vi "Media整体图.vi"() -> ()   [LabVIEW 2014]
panel:
  in  "Mute":bool
  in  "Music":bool
  in  "Multimedia":bool
  in  "Mix":bool
  in  "Mediaplayer":bool
  in  "Jukebox":bool
  in  "Ipod":bool
  in  "Dvd":bool
  in  "Create":bool
  in  "Control":bool
  in  "Chat":bool
  in  "Cdwriter":bool
  in  "Cdrom":bool
  in  "Cd":bool
  in  "Camera":bool
  in  "Build":bool
  in  "Bell":bool
  in  "Audio cd":bool
  in  "Arts":bool
  in  "Action":bool
  in  "Volume":bool
  in  "Unknown":bool
  in  "Tv":bool
  in  "Sound":bool
  in  "Snap":bool
  in  "Record volume":bool
  in  "Realplayer":bool
  in  "Player":bool
  in  "Play":bool
  in  "Piano":bool
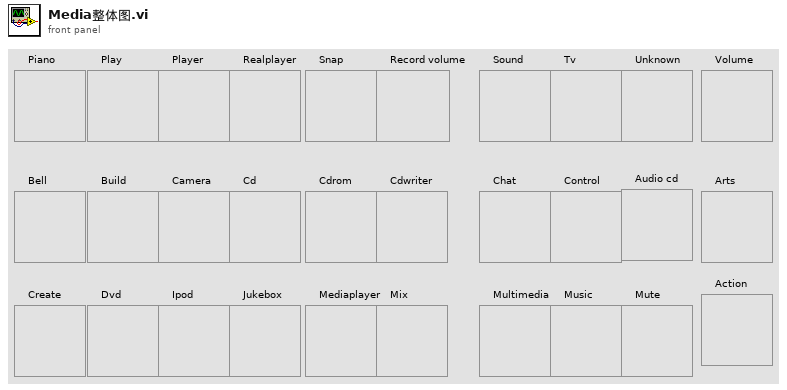
[diagram p1: front panel]
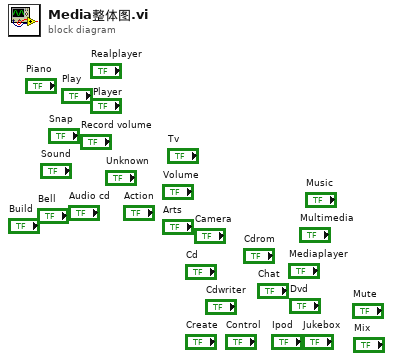
[diagram p0: block diagram]
diagram:
